vi "create.ModifyOrderLong.vi"(8 "error in":errorcluster, 10 "ModifyOrderLong.Parameters":T1, 11 "ModifyOrderLong in":refnum<class "ModifyOrderLong.lvclass">) -> (0 "error out":errorcluster, 3 "ModifyOrderLong out":refnum<class "ModifyOrderLong.lvclass">)   [LabVIEW 2022 SP3, in "ModifyOrderLong.lvclass"]
uses:
  ModifyOrderLong.lvclass
  ModifyOrderLong.Parameters.ctl
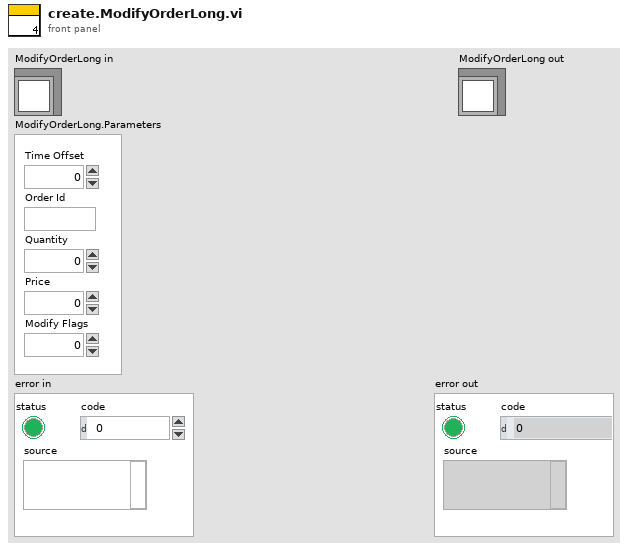
[diagram p1: front panel]
types:
  T1 = typedef "ModifyOrderLong.lvclass/ModifyOrderLong.Parameters.ctl" = cluster{"Time Offset":u32, "Order Id":string, "Quantity":u32, "Price":dbl, "Modify Flags":u8}
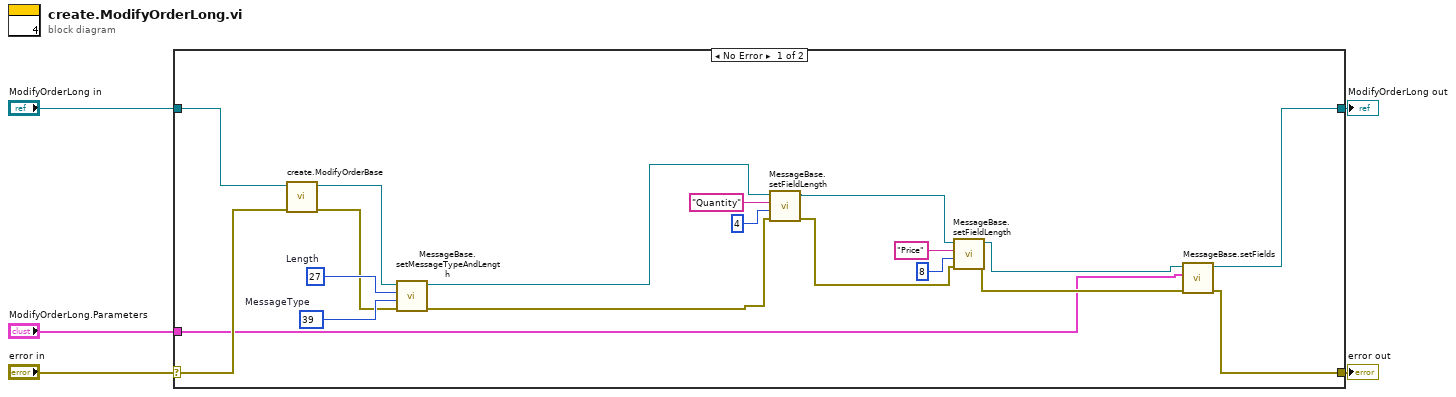
[diagram p0: block diagram]
diagram:
  n1 = case shown="No Error" "error in" {
    selector: "error in" -> [w23 w26]
    tunnel: [w8 w26] -> w4
    tunnel: [w7 w25] -> w2
    tunnel: "ModifyOrderLong in" -> [w24 w25]
    tunnel: "ModifyOrderLong.Parameters" -> [w6 _]
    frame No Error {
      w21 = u8 39  # MessageType
      w22 = u8 27  # Length
      n2 = call-dynamic "create.ModifyOrderBase.vi"("error in (no error)"=w23, "ModifyOrderBase in"=w24) -> ("error out"=w19:errorcluster, "ModifyOrderBase out"=w20:refnum<class "ModifyOrderLong.lvclass">)  [unwired: 8 in]
      n3 = call-dynamic "MessageBase.setMessageTypeAndLength.vi"("error in (no error)"=w19, "MessageType"=w21, "Length"=w22, "MessageBase in"=w20) -> ("error out"=w11:errorcluster, "MessageBase out"=w12:refnum<class "ModifyOrderLong.lvclass">)  [unwired: 6 in]
      n4 = call-dynamic "MessageBase.setFieldLength.vi"("error in (no error)"=w11, "Length"=4, "FIeld.Name"="Quantity" ("Field.Name"), "MessageBase in"=w12) -> ("error out"=w13:errorcluster, "MessageBase out"=w14:refnum<class "ModifyOrderLong.lvclass">)  [unwired: 6 in]
      n5 = call-dynamic "MessageBase.setFieldLength.vi"("error in (no error)"=w13, "Length"=8, "FIeld.Name"="Price" ("Field.Name"), "MessageBase in"=w14) -> ("error out"=w9:errorcluster, "MessageBase out"=w10:refnum<class "ModifyOrderLong.lvclass">)  [unwired: 6 in]
      n6 = call-dynamic "MessageBase.setFields.vi"("error in (no error)"=w9, "Cluster (dup)"=w6, "MessageBase in"=w10) -> ("error out"=w8:errorcluster, "MessageBase out"=w7:refnum<class "ModifyOrderLong.lvclass">)  [unwired: 7 in]
    }
    frame Error {
    }
  }
  "error out" <- w4
  "ModifyOrderLong out" <- w2
